vi "onTestExecution.vi"(6 "timeout (2000 ms)":i32=2000, 7 "Name":string, 8 "error in (no error)":errorcluster, 11 "Test Runner.JUnit in":refnum<class "Test Runner.JUnit.lvclass">) -> (0 "error out":errorcluster, 3 "Test Runner.JUnit out":refnum<class "Test Runner.JUnit.lvclass">)   [LabVIEW 2020, in "Test Runner.JUnit.lvclass"]
uses:
  Test Runner.JUnit.lvclass
  classes/Test/Test.lvclass
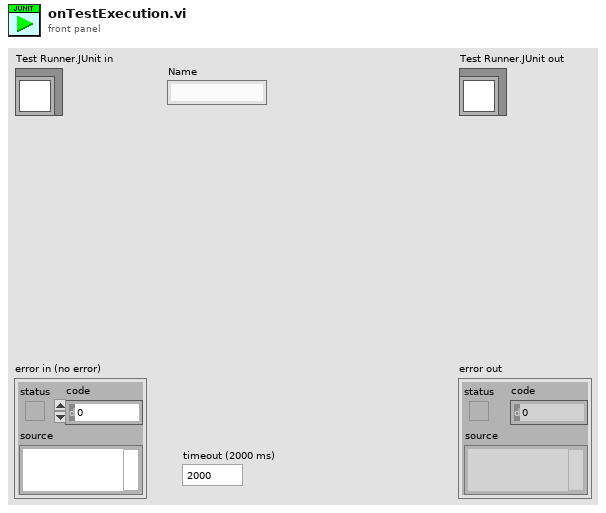
[diagram p1: front panel]
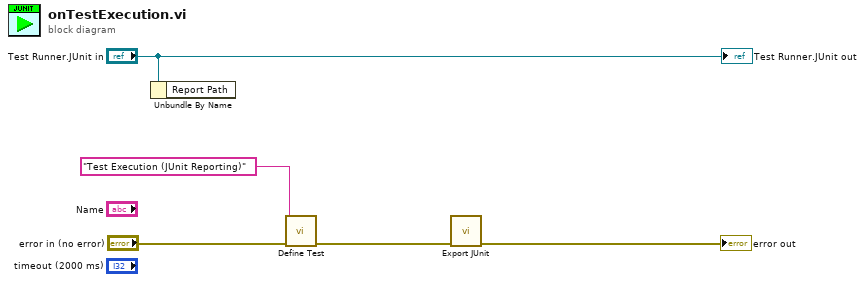
[diagram p0: block diagram]
diagram:
  n1 = Unbundle By Name("Test Runner.JUnit in") -> ()  [unwired: 1 out]
  n2 = call "Define Test.vi"("error in (no error)"="error in (no error)", "Label (VI Title)"="Test Execution (JUnit Reporting)") -> ("error out"=w2:errorcluster)  [unwired: 8 in, 1 out]
  n3 = call "Export JUnit.vi"("error in (no error)"=w2) -> ("error out"=→"error out":errorcluster)  [unwired: 10 in]
  "Test Runner.JUnit out" <- "Test Runner.JUnit in"
